vi "locate files.vi"(8 "error in":errorcluster, 11 "vi modification tool in":refnum<class "vi modification tool.lvclass">) -> (0 "error out":errorcluster, 3 "vi modification tool out":refnum<class "vi modification tool.lvclass">)   [LabVIEW 2013, in "vi modification tool.lvclass"]
uses:
  vi modification tool.lvclass
  vi modification tool.lvclass/vi modification tool.ctl
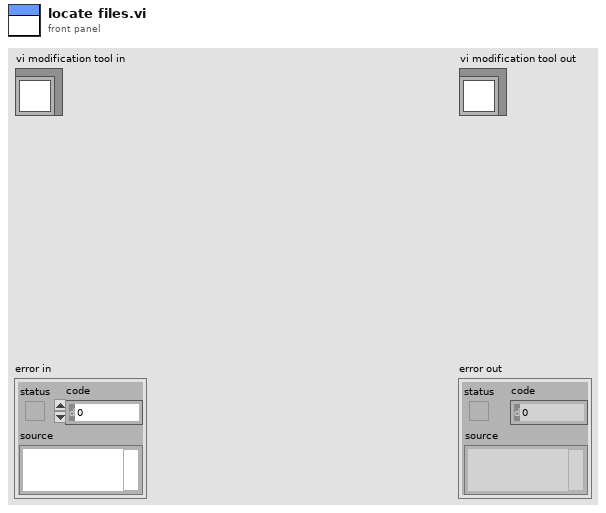
[diagram p1: front panel]
types:
  T1 = typedef "vi modification tool.lvclass/search paths.ctl" = cluster{"Path":path, "exclusions":string[], "include llb":bool}
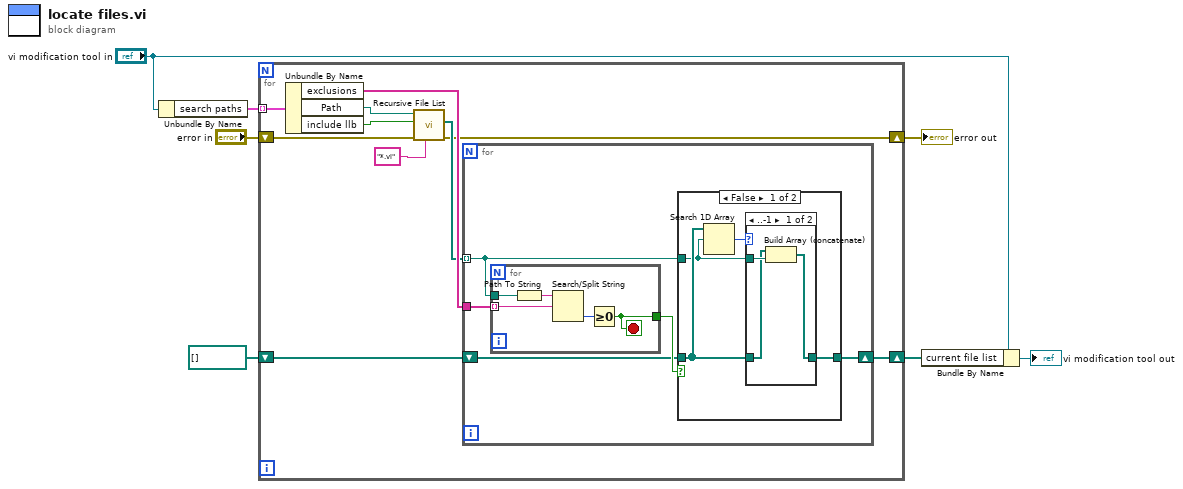
[diagram p0: block diagram]
diagram:
  n1 = Unbundle By Name("vi modification tool in") -> ("search paths"=w7:T1[])
  n2 = for {
    tunnel: w7 -> [w17] mode=indexing
    shift-right: [w11] -> w2
    shift-left: "error in" -> [w14]
    shift-right: [w9] -> w1
    shift-left: path[] [] -> [w10]
    n3 = Unbundle By Name(w17) -> ("exclusions"=w13:string[], "Path"=w16:path, "include llb"=w15:bool)
    n4 = call <vilib>:"Recursive File List.vi"("pattern"="*.vi", "error in (no error)"=w14, "Treat LLBs as Folders?"=w15, "Folder Path"=w16) -> ("error out"=w11:errorcluster, "All Files in Dir"=w12:path[])  [unwired: 3 in, 3 out]
    n5 = for {
      tunnel: w12 -> [w18] mode=indexing
      tunnel: w13 -> [w22]
      shift-right: [w20] -> w9
      shift-left: w10 -> [w19]
      n6 = for {
        tunnel: w18 -> [w32]
        tunnel: w22 -> [w36] mode=indexing
        tunnel: [w34] -> w21
        stop <- w34 stop-if-true
        n7 = Path To String(path=w32) -> (string=w33:string)
        n8 = Search/Split String(string=w33, search string/char (-)=w36) -> (offset of match=w35:i32)  [unwired: 1 in, 2 out]
        n9 = Greater Or Equal To 0?(x=w35) -> (x >= 0?=w34:bool)
      }
      n10 = case shown="False" w21 {
        tunnel: [w25 w31] -> w20
        tunnel: w19 -> [w24 w31]
        tunnel: w18 -> [w23 _]
        frame False {
          n11 = Search 1D Array(1D array=w24, element=w23) -> (index of element=w26:i32)  [unwired: 1 in]
          n12 = case shown="..-1" w26 {
            tunnel: [w27 w30] -> w25
            tunnel: w24 -> [w28 w30]
            tunnel: w23 -> [w29 _]
            frame ..-1 {
              n13 = Build Array (concatenate)(w28, w29) -> (w27:path[])
            }
            frame 0.. {
            }
          }
        }
        frame True {
        }
      }
    }
  }
  "error out" <- w2
  n14 = Bundle By Name(cluster="vi modification tool in", "current file list"=w1) -> (→"vi modification tool out":refnum<class "vi modification tool.lvclass">)
